vi "Read from Property Bag.vi"(8 "error in (no error)":errorcluster, 9 "Data in":variant, 11 "INI Serializer in":refnum<class "INI Serializer.lvclass">) -> (0 "error out":errorcluster, 3 "INI Serializer out":refnum<class "INI Serializer.lvclass">)   [LabVIEW 2014, in "INI Serializer.lvclass"]
uses:
  INI Serializer.lvclass
  INI Serializer.lvclass/INI Serializer.ctl
  <vilib>/Utility/error.llb/Error Cluster From Error Code.vi
  <vilib>/Utility/config.llb/Write Key (Boolean).vi
  <vilib>/Utility/config.llb/Write Key (Double).vi
  <vilib>/Utility/config.llb/Write Key (I32).vi
  <vilib>/Utility/config.llb/Write Key (Path).vi
  <vilib>/Utility/config.llb/Write Key (String).vi
  <vilib>/Utility/config.llb/Write Key (U32).vi
  CI Serializer/CI Serializer.lvclass
  <vilib>/ErrorRing/Error Ring.xnode
  <vilib>/Utility/config.llb/NI_LVConfig.lvlib
  <vilib>/Utility/VariantDataType/VariantType.lvlib
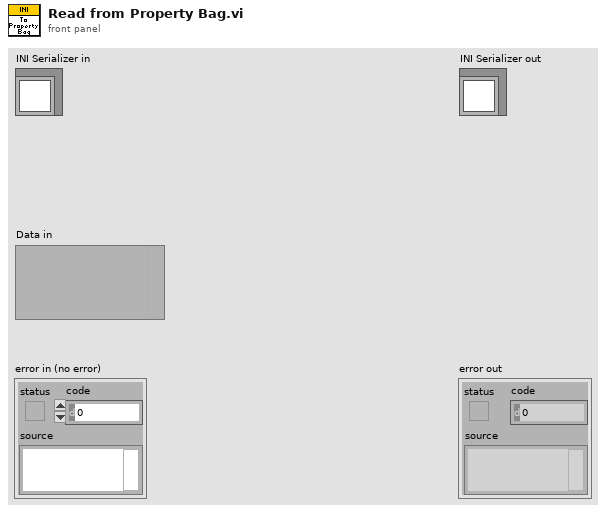
[diagram p1: front panel]
types:
  T1 = typedef "NI_LVConfig.lvlib/Config Data RefNum.ctl" = refnum<k1>
  T2 = typedef "VariantType.lvlib/Type.ctl" = enum8{"Invalid Type", "Void", "I8", "I16", "I32", "I64", "U8", "U16", "U32", "U64", "Single Float", "Double Float", "Extended Float", "Single Complex", "Double Complex", "Extended Complex", "Enum U8", "Enum U16", "Enum U32", "Enum U64", "Single Float With Unit", "Double Float With Unit", "Extended Float With Unit", "Single Complex with Unit", "Double Complex with Unit", "Extended Complex with Unit", "Boolean", "String", "Path", "Picture", "Tag", "Array", "Cluster", "Variant", "LV Variant", "Waveform", "Timestamp", "Digital Waveform", "Digital Data", "ExpressData", "Refnum", "External Data", "VI", "Poly VI", "LabVIEW Class Instance", "Fixed Point"}
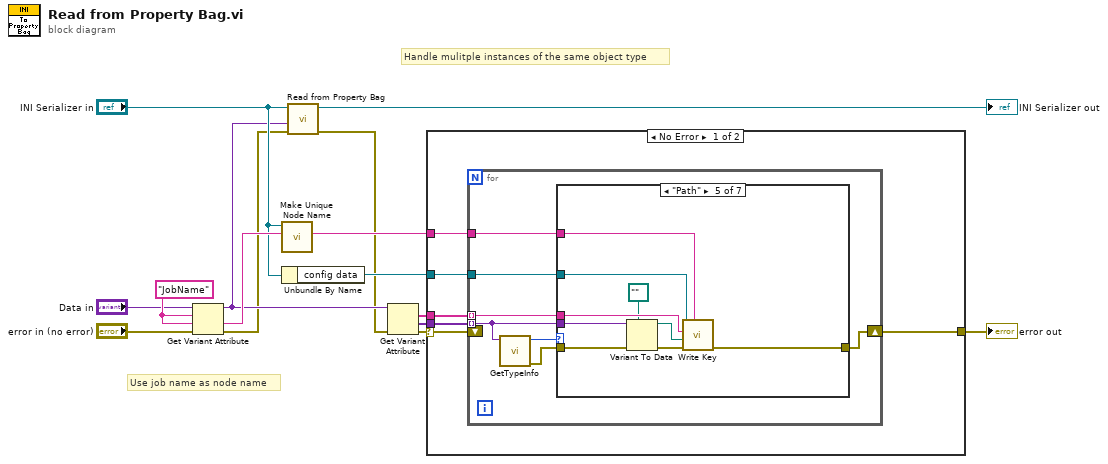
[diagram p0: block diagram]
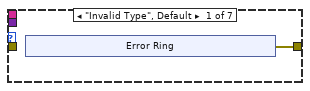
[diagram p2: hidden frame]
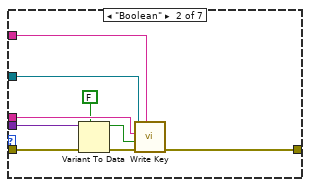
[diagram p3: hidden frame]
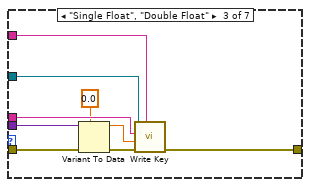
[diagram p4: hidden frame]
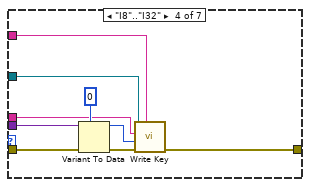
[diagram p5: hidden frame]
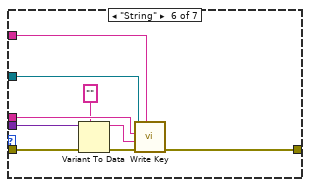
[diagram p6: hidden frame]
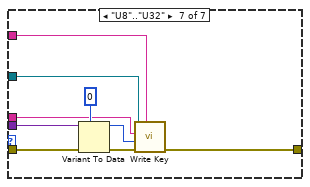
[diagram p7: hidden frame]
diagram:
  w9 = "JobName" ("name")
  # "Use job name as node name"
  # "Handle mulitple instances of the same object type"
  n1 = Get Variant Attribute(Variant="Data in", name=w9, default value (empty Variant)=w9, error in="error in (no error)") -> (duplicate Variant=w4:variant, value=w6:string, error out=w3:errorcluster)  [unwired: 1 out]
  n2 = call "Make Unique Node Name.vi"("Node Name"=w6, "CI Serializer in"="INI Serializer in") -> ("Unique Node Name"=w10:string)  [unwired: 9 in]
  n3 = Unbundle By Name("INI Serializer in") -> ("config data"=w14:T1)
  n4 = call-parent "Read from Property Bag.vi"("error in (no error)"=w3, "Data in"=w4, "CI Serializer in"="INI Serializer in") -> ("error out"=w2:errorcluster, "CI Serializer out"=→"INI Serializer out":refnum<class "INI Serializer.lvclass">)  [unwired: 7 in]
  n5 = Get Variant Attribute(Variant=w4, error in=w2) -> (names=w13:string[], values=w15:variant[], error out=w12:errorcluster)  [unwired: 2 in, 1 out]
  n6 = case shown="No Error" w12 {
    selector: w12 -> [w19 w88]
    tunnel: w15 -> [w21 _]
    tunnel: w14 -> [w16 _]
    tunnel: w10 -> [w17 _]
    tunnel: w13 -> [w20 _]
    tunnel: [w18 w88] -> w11
    frame No Error {
      n7 = for {
        tunnel: w21 -> [w27] mode=indexing
        tunnel: w16 -> [w26]
        tunnel: w17 -> [w25]
        tunnel: w20 -> [w24] mode=indexing
        shift-right: [w22] -> w18
        shift-left: w19 -> [_]
        n8 = call <vilib>:"GetTypeInfo.vi"("Variant"=w27) -> ("error out"=w23:errorcluster, "Type Enum"=w28:T2)  [unwired: 6 in, 3 out]
        n9 = case shown="\"Path\"" w28 {
          tunnel: w27 -> [_ w41 w50 w58 w68 w77 w85]
          tunnel: w26 -> [_ w39 w48 w56 w66 w75 w83]
          tunnel: w25 -> [_ w38 w47 w55 w65 w74 w82]
          tunnel: w24 -> [_ w37 w46 w54 w64 w73 w81]
          tunnel: w23 -> [_ w35 w44 w53 w62 w71 w79]
          tunnel: [w29 w34 w43 w52 w61 w70 w80] -> w22
          frame "Invalid Type", Default {
            n10 = xnode "Error Ring"() -> ("error out"=w29:errorcluster)
          }
          frame "Boolean" {
            n11 = Variant To Data(error in=w35, type=FALSE, Variant=w41) -> (data=w42:bool, error out=w40:errorcluster)
            n12 = call-poly <vilib>:"Write Key.vi"("section"=w38, "error in (no error)"=w40, "value"=w42, "key"=w37, "refnum"=w39) -> ("error out"=w34:errorcluster)  [unwired: 4 in, 2 out]
          }
          frame "Single Float", "Double Float" {
            n13 = Variant To Data(error in=w44, type=0.0, Variant=w50) -> (data=w51:dbl, error out=w49:errorcluster)
            n14 = call-poly <vilib>:"Write Key.vi"("section"=w47, "error in (no error)"=w49, "value"=w51, "key"=w46, "refnum"=w48) -> ("error out"=w43:errorcluster)  [unwired: 4 in, 2 out]
          }
          frame "I8".."I32" {
            n15 = Variant To Data(error in=w53, type=0 ("value"), Variant=w58) -> (data=w59:i32, error out=w57:errorcluster)
            n16 = call-poly <vilib>:"Write Key.vi"("section"=w55, "error in (no error)"=w57, "value"=w59, "key"=w54, "refnum"=w56) -> ("error out"=w52:errorcluster)  [unwired: 4 in, 2 out]
          }
          frame "Path" {
            n17 = Variant To Data(error in=w62, type=path "", Variant=w68) -> (data=w69:path, error out=w67:errorcluster)
            n18 = call-poly <vilib>:"Write Key.vi"("section"=w65, "error in (no error)"=w67, "value"=w69, "key"=w64, "refnum"=w66) -> ("error out"=w61:errorcluster)  [unwired: 4 in, 2 out]
          }
          frame "String" {
            n19 = Variant To Data(error in=w71, type="", Variant=w77) -> (data=w78:string, error out=w76:errorcluster)
            n20 = call-poly <vilib>:"Write Key.vi"("section"=w74, "error in (no error)"=w76, "value"=w78, "key"=w73, "refnum"=w75) -> ("error out"=w70:errorcluster)  [unwired: 4 in, 2 out]
          }
          frame "U8".."U32" {
            n21 = Variant To Data(error in=w79, type=u32 0 ("value"), Variant=w85) -> (data=w86:u32, error out=w84:errorcluster)
            n22 = call-poly <vilib>:"Write Key.vi"("section"=w82, "error in (no error)"=w84, "value"=w86, "key"=w81, "refnum"=w83) -> ("error out"=w80:errorcluster)  [unwired: 4 in, 2 out]
          }
        }
      }
    }
    frame Error {
    }
  }
  "error out" <- w11
